vi "Test Get Table Rows by Column Value (VAR).vi"(11 "Test Case In":refnum<class "Test Open Xml.lvclass">) -> (0 "error out":errorcluster, 3 "Test Case Out":refnum<class "Test Open Xml.lvclass">)   [LabVIEW 2020, in "Test Open Xml.lvclass"]
uses:
  Test Open Xml.lvclass
  Test Open Xml.lvclass/Test Open Xml.ctl
  Source/Open Xml.lvlib
  0a0d70f3-36fe-46ba-8b3e-e6c07e708d9f.vi
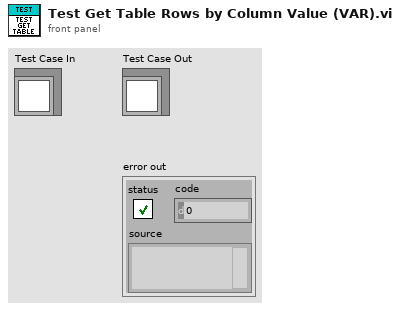
[diagram p1: front panel]
types:
  T1 = cluster{"Sheet Name":string, "Name":string, "Display Name":string, "Range":string}
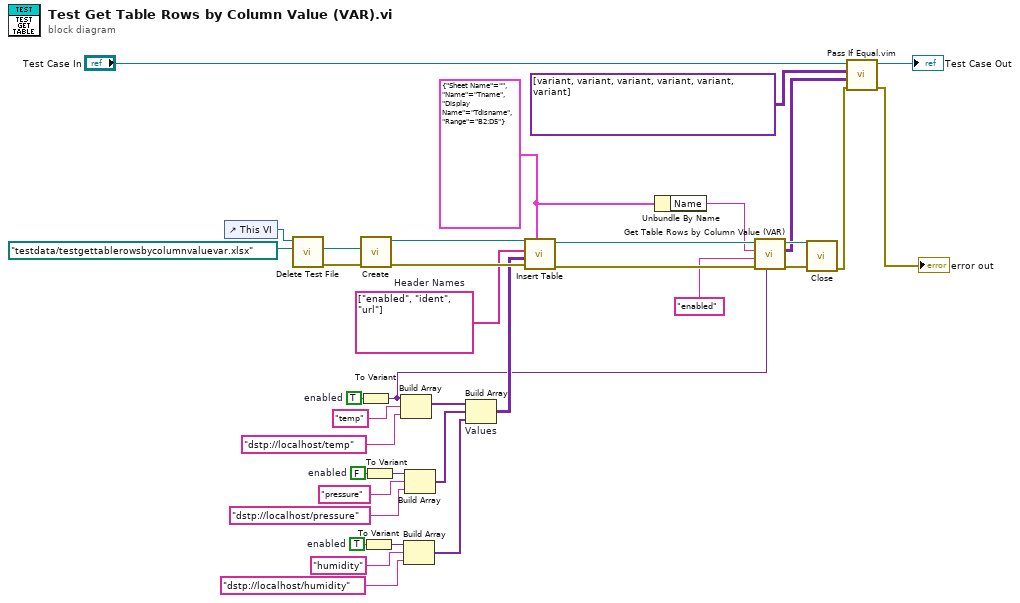
[diagram p0: block diagram]
diagram:
  w10 = TRUE  # enabled
  w18 = FALSE  # enabled
  w24 = TRUE  # enabled
  w25 = string[] ["enabled", "ident", "url"]  # Header Names
  w5 = T1 {"Sheet Name"="", "Name"="Tname", "Display Name"="Tdisname", "Range"="B2:D5"} ("Location")
  n1 = control-ref of="This VI"() -> (w29:refnum<vi>)
  n2 = call "Delete Test File.vi"("name or relative path"=path "testdata/testgettablerowsbycolumnvaluevar.xlsx", "VI in"=w29) -> ("error out"=w30:errorcluster, "deleted path"=w31:path)  [unwired: 8 in]
  n3 = call "Create.vi"("error in"=w30, "Path"=w31) -> ("error out"=w26:errorcluster, "SpreadsheetDoc"=w27:refnum<k24>)  [unwired: 8 in]
  n4 = To Variant(anything=w24) -> (Variant=w3:variant)
  n5 = To Variant(anything=w10) -> (Variant=w9:variant)
  n6 = To Variant(anything=w18) -> (Variant=w19:variant)
  n7 = Build Array(w3, "temp", "dstp://localhost/temp") -> (w17:variant[])
  n8 = Build Array(w9, "humidity", "dstp://localhost/humidity") -> (w6:variant[])
  n9 = Build Array(w19, "pressure", "dstp://localhost/pressure") -> (w16:variant[])
  n10 = Build Array "Values"(w17, w16, w6) -> (w12:variant[][])
  n11 = call "Insert Table.vi"("Location"=w5, "error in"=w26, "Cell Values"=w12, "Header Names"=w25, "SpreadsheetDoc in"=w27) -> ("error out"=w32:errorcluster, "SpreadsheetDoc out"=w14:refnum<k24>)  [unwired: 5 in]
  n12 = Unbundle By Name(w5) -> ("Name"=w4:string)
  n13 = call "Get Table Rows by Column Value (VAR).vi"("Column Value"=w3, "error in"=w32, "Column Name"="enabled", "Table Name"=w4, "SpreadsheetDoc in"=w14) -> ("error out"=w15:errorcluster, "Cell Values"=w11:variant[][], "SpreadsheetDoc out"=w13:refnum<k24>)  [unwired: 4 in]
  n14 = call "Close.vi"("error in"=w15, "SpreadsheetDoc"=w13) -> ("error out"=w33:errorcluster)  [unwired: 9 in]
  n15 = call "Pass If Equal.vim"("error in (no error)"=w33, "Actual"=w11, "Expected"=variant[][] [[variant(bool TRUE), variant(string "temp"), variant(string "dstp://localhost/temp")], [variant(bool TRUE), variant(string "humidity"), variant(string "dstp://localhost/humidity")]] ("Cell Values"), "LUnit Test Case In"="Test Case In") -> ("error out"=→"error out":errorcluster, "LUnit Test Case Out"=→"Test Case Out":refnum<class "Test Open Xml.lvclass">)  [unwired: 6 in]
